vi "Initialize Parameter Manager.vi"(8 "error in (no error)":errorcluster, 10 "VI Refnum":refnum<vi>, 11 "CD Item Ref":u64) -> (0 "error out":errorcluster, 3 "CD Parameter Manager out":refnum<class "CD Parameter Manager.lvclass">)   [LabVIEW 2019, in "CD Parameter Manager API.lvlib" / "CD Parameter Manager.lvclass"]
uses:
  CD Parameter Manager.lvclass
  CD Parameter Manager.lvclass/CD Parameter Manager.ctl
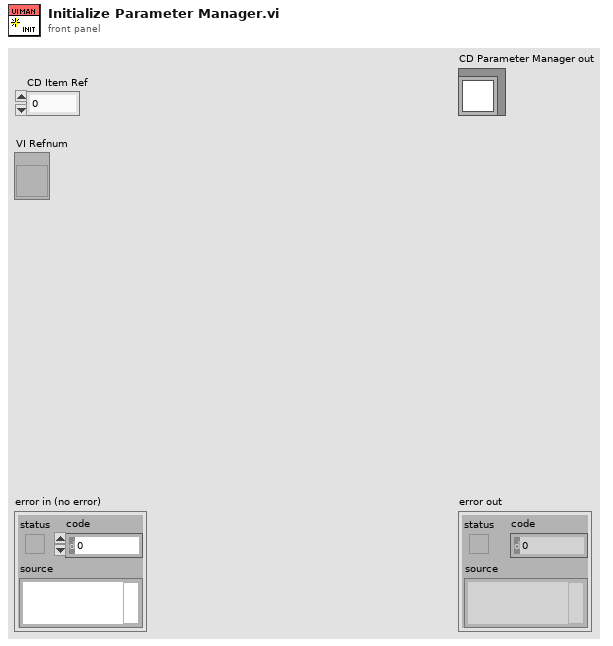
[diagram p1: front panel]
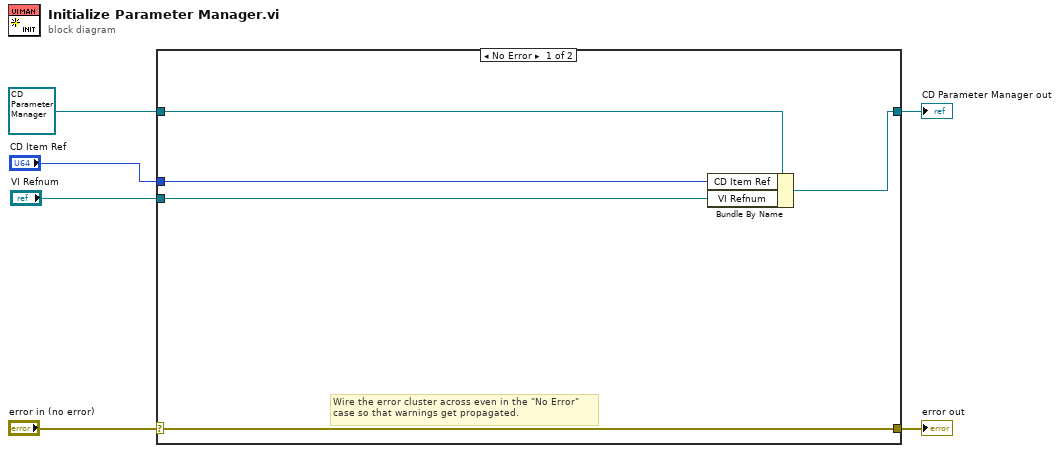
[diagram p0: block diagram]
diagram:
  n1 = case shown="No Error" "error in (no error)" {
    selector: "error in (no error)" -> [w11 w13]
    tunnel: [w11 w13] -> w5
    tunnel: [w8 w12] -> w3
    tunnel: refnum<class "CD Parameter Manager.lvclass"> refnum ("CD Parameter Manager in") -> [w10 w12]
    tunnel: "VI Refnum" -> [w9 _]
    tunnel: "CD Item Ref" -> [w7 _]
    frame No Error {
      # "Wire the error cluster across even in the \"No Error\"\ncase so that warnings get propagated."
      n2 = Bundle By Name(cluster=w10, "CD Item Ref"=w7, "VI Refnum"=w9) -> (w8:refnum<class "CD Parameter Manager.lvclass">)
    }
    frame Error {
    }
  }
  "error out" <- w5
  "CD Parameter Manager out" <- w3
